vi "storeADCMixedToArray-wang-test2simplified2.vi"(0 "String":string) -> (18 "Graph Data":T1)   [LabVIEW 2014]
uses:
  main/controls/Graph Data.ctl
  <vilib>/Utility/miscctls.llb/LVAnnotationListTypeDef.ctl
  <vilib>/Utility/miscctls.llb/LVCursorListTypeDef.ctl
  main/global/Global ADCarray.vi
panel:
  out "Array - Numeric":i32[](array[numeric])
  out "CH7":i32[](array[numeric])
  out "CH6":i32[](array[numeric])
  out "CH5":i32[](array[numeric])
  out "CH4":i32[](array[numeric])
  out "CH3":i32[](array[numeric])
  out "CH2":i32[](array[numeric])
  out "CH1":i32[](array[numeric])
  out "CH0":i32[](array[numeric])
  out "Array - String":string[](array[string])
  out "Number of channel":u8[](array[numeric])
  out "Waveform":waveform(dbl)
  out "Graph":waveform(i32)[](graph)
  out "Numeric 2":i32
  out "Nombre de pixel":i32
  out "TotalTrigger":i32
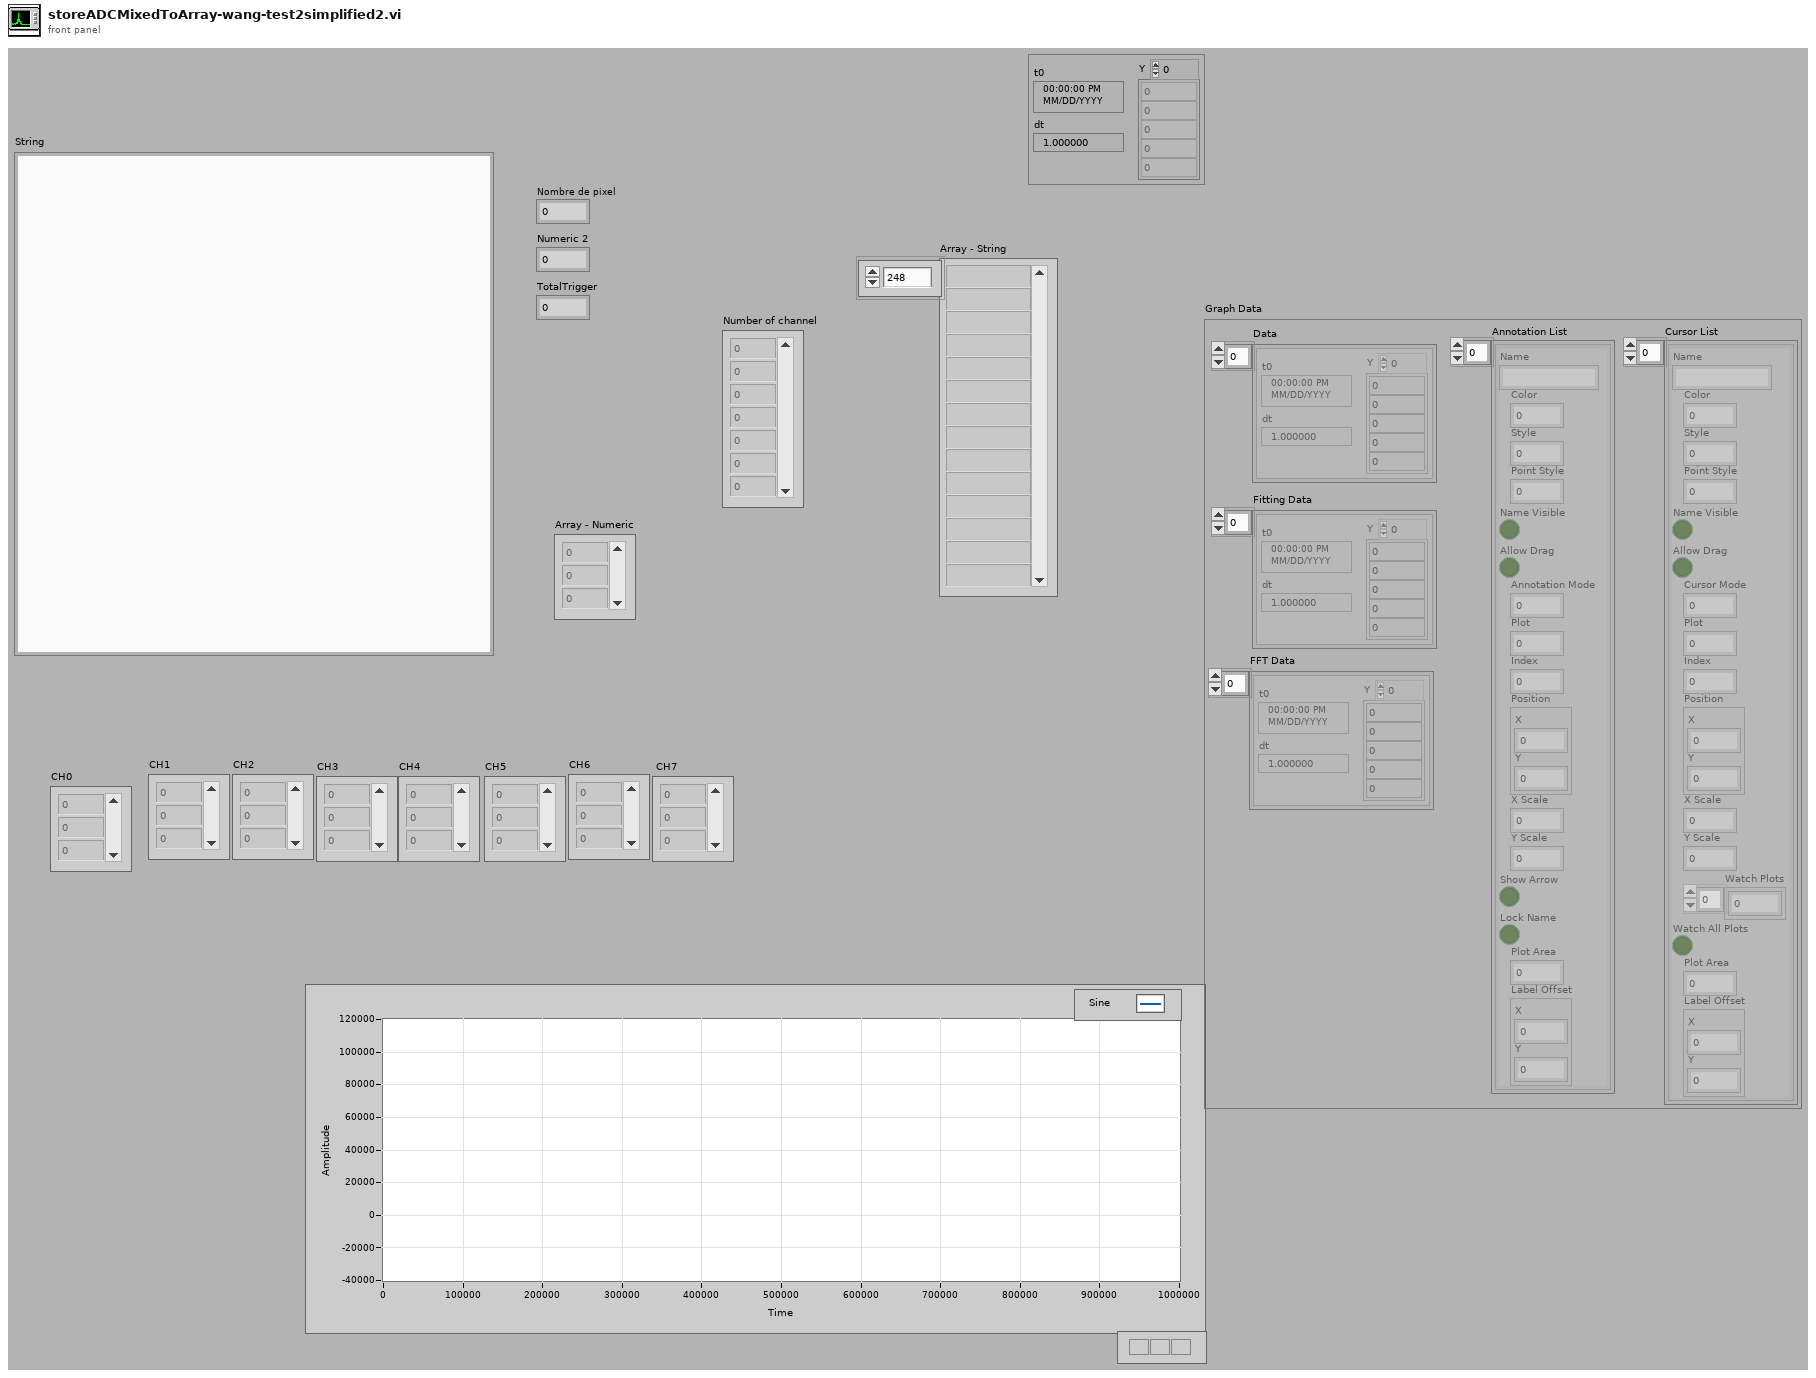
[diagram p1: front panel]
types:
  T1 = typedef "Graph Data.ctl" = cluster{"Data":waveform(dbl)[], "Annotation List":T2, "Cursor List":T3, "Fitting Data":waveform(dbl)[], "FFT Data":waveform(dbl)[]}
  T2 = typedef "LVAnnotationListTypeDef.ctl" = cluster{"Name":string, "Color":u32, "Style":u8, "Point Style":u8, "Name Visible":bool, "Allow Drag":bool, "Annotation Mode":u32, "Plot":i32, "Index":i32, "Position":cluster{"X":dbl, "Y":dbl}, "X Scale":u32, "Y Scale":u32, "Show Arrow":bool, "Lock Name":bool, "Plot Area":i32, "Label Offset":cluster{"X":dbl, "Y":dbl}}[]
  T3 = typedef "LVCursorListTypeDef.ctl" = cluster{"Name":string, "Color":u32, "Style":u8, "Point Style":u8, "Name Visible":bool, "Allow Drag":bool, "Cursor Mode":u32, "Plot":i32, "Index":i32, "Position":cluster{"X":dbl, "Y":dbl}, "X Scale":u32, "Y Scale":u32, "Watch Plots":i32[], "Watch All Plots":bool, "Plot Area":i32, "Label Offset":cluster{"X":dbl, "Y":dbl}}[]
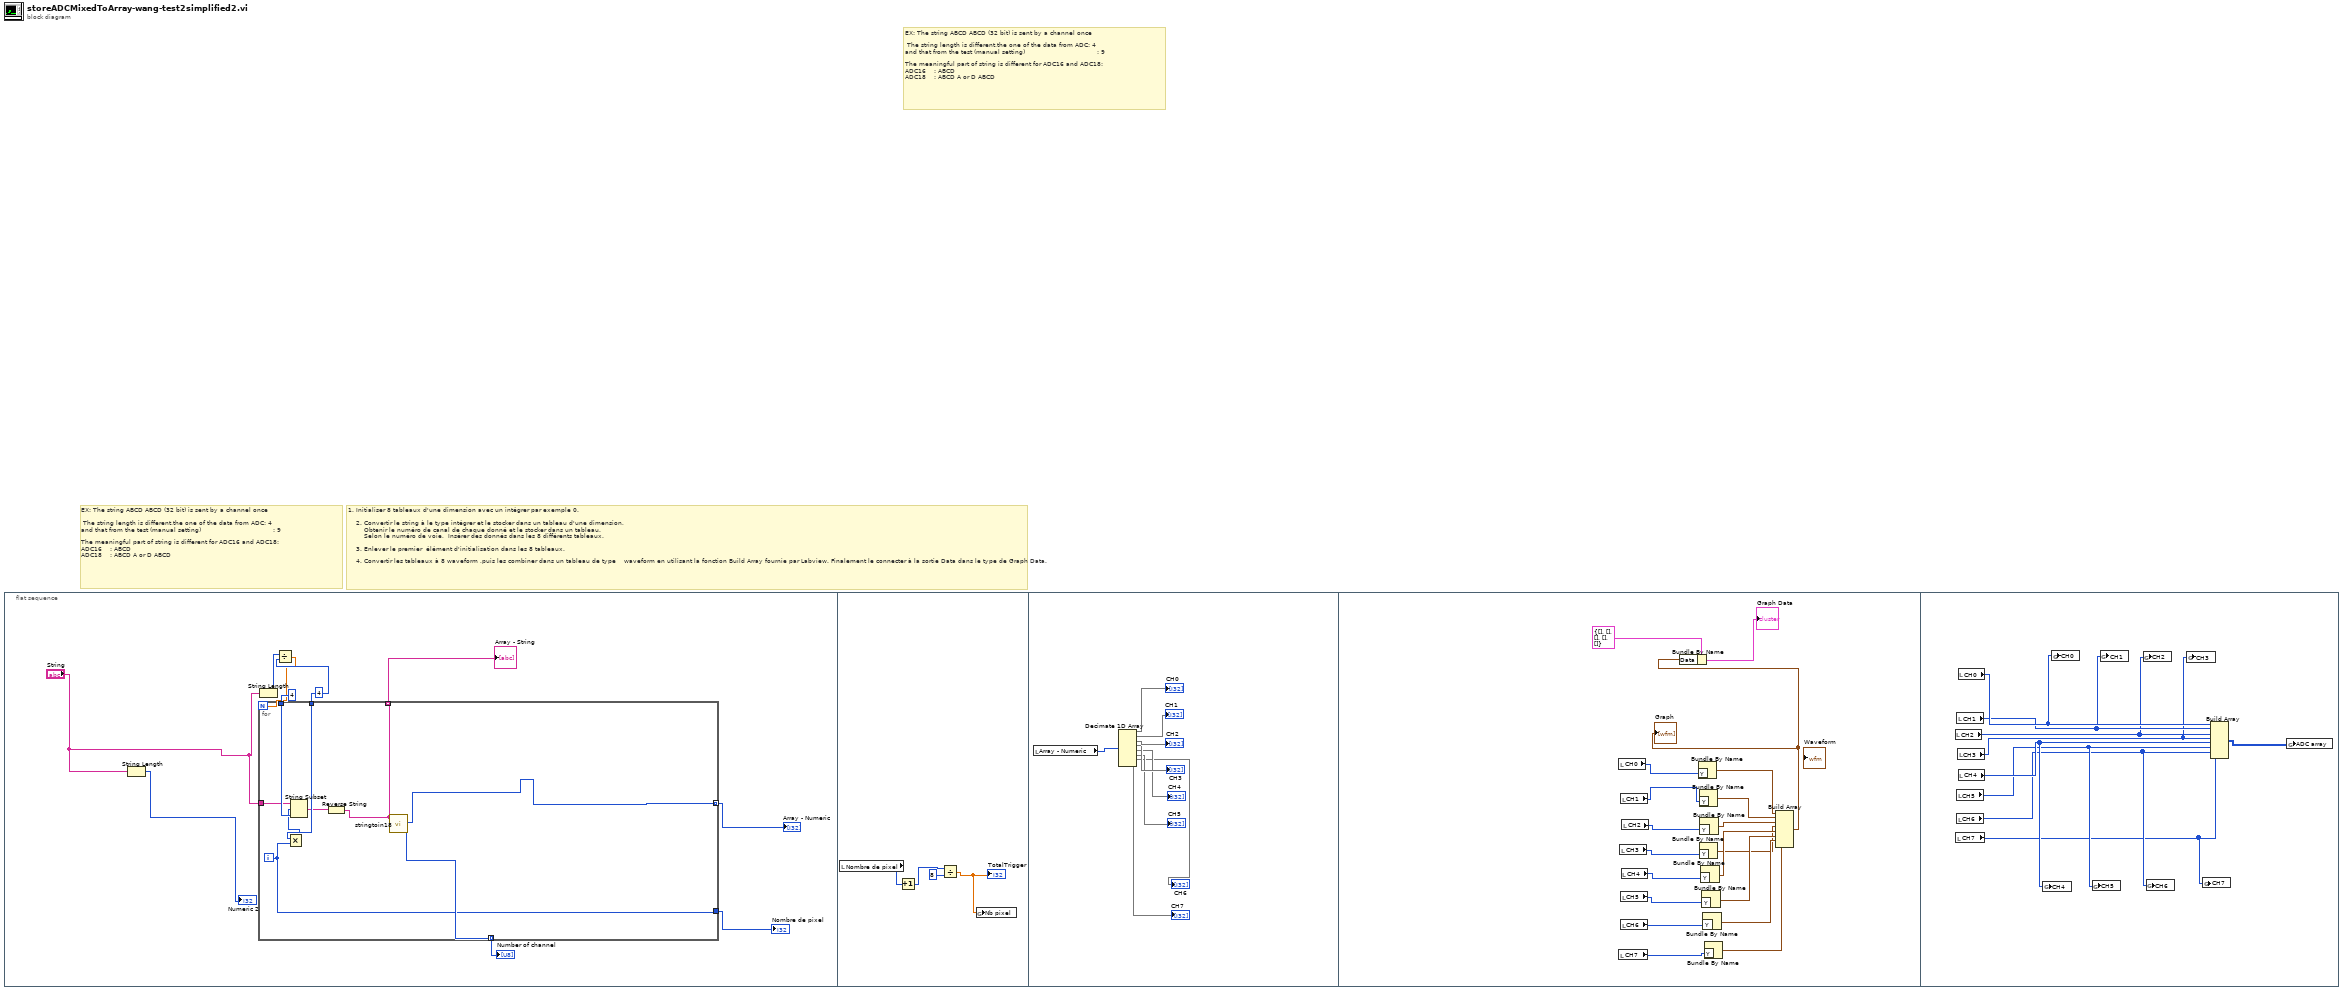
[diagram p0: block diagram]
diagram:
  # "1. Initialiser 8 tableaux d'une dimension avec un intégrer par exemple 0.\n\n    2.\tConvertir le string à le type intégrer et le stocker dans un tableau d'une dimension,\n        Obtenir le numéro de canal de chaque donné et le stocker dans un tableau.  \n        Selon le numéro de voie,  Insérer des donnés dans les 8 différents tableaux.\n\n    3. Enlever le premier  élément d'initialisation dans les 8 tableaux.\n\n    4. Convertir les tableaux à 8 waveform ,puis les combiner dans un tableau de type    waveform en utilisant la fonction Build Array fournie par Labview. Finalement le connecter à la sortie Data dans le type de Graph Data."
  # "EX: The string ABCD ABCD (32 bit) is sent by a channel once                \n\n The string length is different,the one of the data from ADC: 4\nand that from the test (manual setting)                                    : 9\n\nThe meaningful part of string is different for ADC16 and ADC18:\nADC16    : ABCD                          \nADC18    : ABCD A or D ABCD"
  # "EX: The string ABCD ABCD (32 bit) is sent by a channel once                \n\n The string length is different,the one of the data from ADC: 4\nand that from the test (manual setting)                                    : 9\n\nThe meaningful part of string is different for ADC16 and ADC18:\nADC16    : ABCD                          \nADC18    : ABCD A or D ABCD"
  n1 = flat-sequence {
    frame #0 {
      w8 = 4
      n2 = String Length(string="String") -> (length=→"Numeric 2":i32)
      n3 = String Length(string="String") -> (length=w3:i32)
      n4 = Divide(x=w3, y=w8) -> (x/y=w7:dbl)
      n5 = for {
        N: w7 -> [_]
        tunnel: 4 -> [w19]
        tunnel: w8 -> [w18]
        tunnel: [w12] -> w1
        tunnel: "String" -> [w15]
        tunnel: [w14] -> w6 mode=indexing
        tunnel: [w13] -> w5 mode=indexing
        tunnel: [w11] -> w4 mode=indexing
        i -> [w12]
        n6 = Multiply(x=w18, y=w12) -> (x*y=w17:i32)
        n7 = String Subset(string=w15, offset (0)=w17, length (rest)=w19) -> (substring=w16:string)
        n8 = Reverse String(1:w16) -> (0:w13:string)
        n9 = call "stringtoin18.vi"("input_string"=w13) -> ("channel"=w14:u8, "outputComplemented_int"=w11:i32)  [unwired: 7 in, 2 out]
      }
      "Nombre de pixel" <- w1
      "Number of channel" <- w6
      "Array - String" <- w5
      "Array - Numeric" <- w4
    }
    frame #1 {
      n10 = local read "Nombre de pixel"() -> (w23:i32)
      n11 = Increment(x=w23) -> (x+1=w22:i32)
      n12 = Divide(x=w22, y=8) -> (x/y=w20:dbl)
      "TotalTrigger" <- w20
      n13 = global write "Global ADCarray.vi" "Nb pixel"(w20) -> ()
    }
    frame #2 {
      n14 = local read "Array - Numeric"() -> (w24:i32[])
      n15 = Decimate 1D Array(w24) -> (→"CH0":i32[], →"CH1":i32[], →"CH2":i32[], →"CH3":i32[], →"CH4":i32[], →"CH5":i32[], →"CH6":i32[], →"CH7":i32[])
    }
    frame #3 {
      n16 = local read "CH0"() -> (w33:i32[])
      n17 = local read "CH7"() -> (w37:i32[])
      n18 = local read "CH3"() -> (w41:i32[])
      n19 = local read "CH1"() -> (w35:i32[])
      n20 = local read "CH5"() -> (w39:i32[])
      n21 = local read "CH6"() -> (w38:i32[])
      n22 = local read "CH4"() -> (w40:i32[])
      n23 = local read "CH2"() -> (w42:i32[])
      n24 = Bundle By Name("Y"=w33) -> (w34:waveform(i32))  [unwired: 1 in]
      n25 = Bundle By Name("Y"=w35) -> (w36:waveform(i32))  [unwired: 1 in]
      n26 = Bundle By Name("Y"=w41) -> (w44:waveform(i32))  [unwired: 1 in]
      n27 = Bundle By Name("Y"=w42) -> (w43:waveform(i32))  [unwired: 1 in]
      n28 = Bundle By Name("Y"=w40) -> (w48:waveform(i32))  [unwired: 1 in]
      n29 = Bundle By Name("Y"=w39) -> (w45:waveform(i32))  [unwired: 1 in]
      n30 = Bundle By Name("Y"=w38) -> (w46:waveform(i32))  [unwired: 1 in]
      n31 = Bundle By Name("Y"=w37) -> (w47:waveform(i32))  [unwired: 1 in]
      n32 = Build Array(w34, w36, w43, w44, w48, w45, w46, w47) -> (w49:waveform(i32)[])
      "Graph" <- w49
      n33 = Bundle By Name(cluster=T1 {"Data"=[], "Annotation List"=[], "Cursor List"=[], "Fitting Data"=[], "FFT Data"=[]} ("Graph Data"), "Data"=w49) -> (→"Graph Data":T1)
    }
    frame #4 {
      n34 = local read "CH2"() -> (w57:i32[])
      n35 = local read "CH7"() -> (w52:i32[])
      n36 = local read "CH5"() -> (w54:i32[])
      n37 = local read "CH6"() -> (w53:i32[])
      n38 = local read "CH1"() -> (w58:i32[])
      n39 = local read "CH3"() -> (w56:i32[])
      n40 = local read "CH0"() -> (w59:i32[])
      n41 = local read "CH4"() -> (w55:i32[])
      n42 = global write "Global ADCarray.vi" "CH4"(w55) -> ()
      n43 = global write "Global ADCarray.vi" "CH0"(w59) -> ()
      n44 = global write "Global ADCarray.vi" "CH5"(w54) -> ()
      n45 = global write "Global ADCarray.vi" "CH1"(w58) -> ()
      n46 = global write "Global ADCarray.vi" "CH2"(w57) -> ()
      n47 = global write "Global ADCarray.vi" "CH6"(w53) -> ()
      n48 = global write "Global ADCarray.vi" "CH3"(w56) -> ()
      n49 = global write "Global ADCarray.vi" "CH7"(w52) -> ()
      n50 = Build Array(w59, w58, w57, w56, w55, w54, w53, w52) -> (w60:i32[][])
      n51 = global write "Global ADCarray.vi" "ADC array"(w60) -> ()
    }
  }
